vi "Get_Rate.vi"(8 "error in (no error)":errorcluster, 11 "Thorlabs_PM100D in":refnum<class "Thorlabs_PM100D.lvclass">) -> (0 "error out":errorcluster, 2 "Frequency":dbl[unit], 3 "Thorlabs_PM100D out":refnum<class "Thorlabs_PM100D.lvclass">)   [LabVIEW 2020, in "Thorlabs_PM100D.lvclass"]
uses:
  <instrlib>/Classes/Powermeter/Thorlabs_PM100D/Thorlabs_PM100D.lvclass
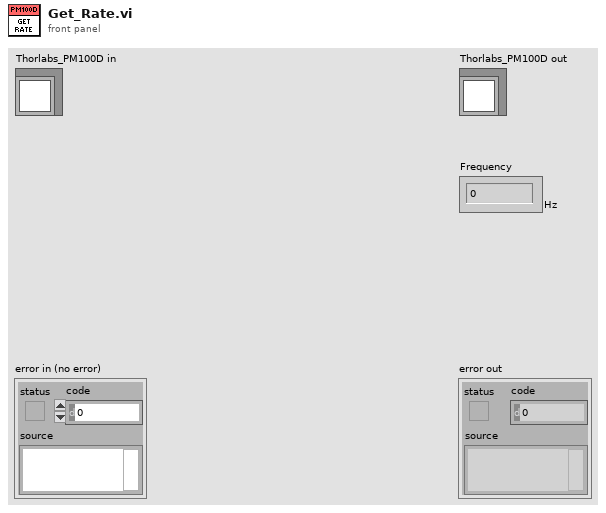
[diagram p1: front panel]
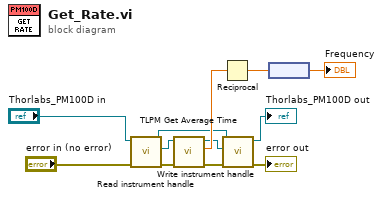
[diagram p0: block diagram]
diagram:
  n1 = call-dynamic "Read instrument handle.vi"("error in (no error)"="error in (no error)", "Thorlabs_PM100D in"="Thorlabs_PM100D in") -> ("error out"=w6:errorcluster, "instrument handle"=w11:refnum<visa-resource-name>, "Thorlabs_PM100D out"=w1:refnum<class "Thorlabs_PM100D.lvclass">)  [unwired: 7 in]
  n2 = call <instrlib>:"TLPM Get Average Time.vi"("error in (no error)"=w6, "instrument handle"=w11) -> ("error out"=w4:errorcluster, "Average Time"=w10:dbl, "instrument handle out"=w3:refnum<visa-resource-name>)  [unwired: 7 in]
  n3 = Reciprocal(x=w10) -> (1/x=w9:dbl)
  n4 = call-dynamic "Write instrument handle.vi"("error in (no error)"=w4, "instrument handle"=w3, "Thorlabs_PM100D in"=w1) -> ("error out"=→"error out":errorcluster, "Thorlabs_PM100D out"=→"Thorlabs_PM100D out":refnum<class "Thorlabs_PM100D.lvclass">)  [unwired: 7 in]
  n5 = node(w9) -> (→"Frequency":dbl[unit])
